vi "Dispense FN - ON - Timer (SubVI).vi"(0 "Settings":T1={"ON Settings"={"Enable Dynamic Setpoint?"=TRUE, "Enable Dynamic Dispense Time?"=TRUE, "Enable Drain Rate Functions"=TRUE, "Dispense Sample Time (s)"=0.1, "Mass Average Samples"=20, "ON Timeout (sec)"=300.0, "1st Setpoint (% of Target)"=90.0, "2nd Setpoint (% of Target)"=95.0, "3rd Setpoint (% of Target)"=100.0, "Measure Dispense Delay (sec)"=10.0, "Minimum Spray Time (s)"=2.0, "Pump Reverse Time (s)"=10.0}, "OFF Settings"={"Drain Sample Time (s)"=0.1, "Drain Rate Ave Size"=100, "Drain Rate Limits (± g/sec)"=100.0, "Level Slope Range (± g/sec)"=0.05, "OFF Timeout (sec)"=300.0, "Near SP Slope Level (± g/sec)"=0.005, "Near Setpoint Threshold (%)"=99.0}, "Overshoot Settings"={"Time Limit (s)"=30.0, "Container MAX (g)"=1500.0, "Max FILL Slope (+/- g/sec)"=100.0, "% Overshot to Enable (>)"=3.0}, "FILL Timeout (s)"=300.0, "Full \nSettle Time (s)"=30.0, "Pre-Hydrate \nSpray Time (s)"=0.0, "Pre-Hydrate \nWait Time (s)"=10.0, "m Value "=1.0, "b Value"=0.0, "Enable Overshoot Adjust?"=FALSE} {"ON Settings"."Pump Reverse Time (s)" min=0.0 max=60.0; "OFF Settings"."Near SP Slope Level (± g/sec)" format="%.3g"; "OFF Settings"."Level Slope Range (± g/sec)" format="%.3g"}, 5 "Reset":bool) -> (14 "Elapsed Time (s)":dbl, 15 "ON Timeout (s)":dbl, 17 "Min Spray Complete?":bool, 18 "Measure Delay Complete?":bool, 19 "Max Spray Complete?":bool)   [LabVIEW 2011]
panel:
  # "ONLY ADJUST\nBOLD VALUES!"
  # "Corrected Mass = SDC Mass * m + b"
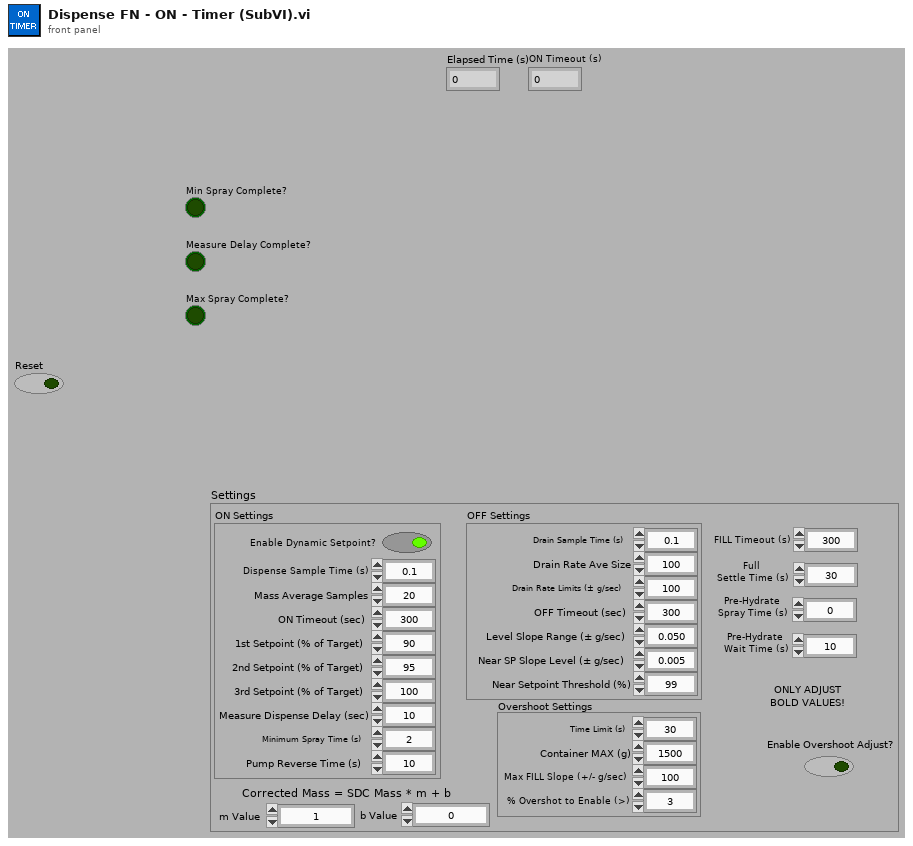
[diagram p1: front panel]
types:
  T1 = cluster{"ON Settings":cluster{"Enable Dynamic Setpoint?":bool, "Enable Dynamic Dispense Time?":bool, "Enable Drain Rate Functions":bool, "Dispense Sample Time (s)":dbl, "Mass Average Samples":i32, "ON Timeout (sec)":dbl, "1st Setpoint (% of Target)":dbl, "2nd Setpoint (% of Target)":dbl, "3rd Setpoint (% of Target)":dbl, "Measure Dispense Delay (sec)":dbl, "Minimum Spray Time (s)":dbl, "Pump Reverse Time (s)":dbl}, "OFF Settings":cluster{"Drain Sample Time (s)":dbl, "Drain Rate Ave Size":i32, "Drain Rate Limits (± g/sec)":dbl, "Level Slope Range (± g/sec)":dbl, "OFF Timeout (sec)":dbl, "Near SP Slope Level (± g/sec)":dbl, "Near Setpoint Threshold (%)":dbl}, "Overshoot Settings":cluster{"Time Limit (s)":dbl, "Container MAX (g)":dbl, "Max FILL Slope (+/- g/sec)":dbl, "% Overshot to Enable (>)":dbl}, "FILL Timeout (s)":dbl, "Full \nSettle Time (s)":dbl, "Pre-Hydrate \nSpray Time (s)":dbl, "Pre-Hydrate \nWait Time (s)":dbl, "m Value ":dbl, "b Value":dbl, "Enable Overshoot Adjust?":bool}
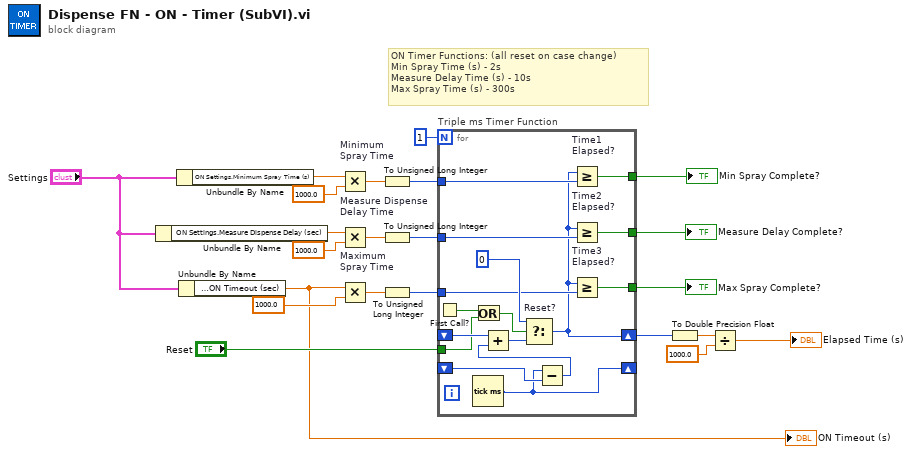
[diagram p0: block diagram]
diagram:
  # "ON Timer Functions: (all reset on case change)\nMin Spray Time (s) - 2s\nMeasure Delay Time (s) - 10s\nMax Spray Time (s) - 300s"
  n1 = Unbundle By Name("Settings") -> ("ON Settings.Measure Dispense Delay (sec)"=w4:dbl)
  n2 = Unbundle By Name("Settings") -> ("ON Settings.Minimum Spray Time (s)"=w3:dbl)
  n3 = Unbundle By Name("Settings") -> ("ON Settings.ON Timeout (sec)"=w5:dbl)
  "ON Timeout (s)" <- w5
  n4 = Multiply "Minimum\nSpray Time"(x=w3, y=1000.0) -> (x*y=w8:dbl)
  n5 = Multiply "Measure Dispense\nDelay Time"(x=w4, y=1000.0) -> (x*y=w13:dbl)
  n6 = Multiply "Maximum\nSpray Time"(x=w5, y=1000.0) -> (x*y=w16:dbl)
  n7 = To Unsigned Long Integer(number=w8) -> (unsigned 32bit integer=w9:u32)
  n8 = To Unsigned Long Integer(number=w13) -> (unsigned 32bit integer=w14:u32)
  n9 = To Unsigned Long Integer(number=w16) -> (unsigned 32bit integer=w17:u32)
  n10 = for "Triple ms Timer Function" {
    N: 1 -> [_]
    shift-right: [w37] -> _
    shift-left: _ -> [w38]
    tunnel: [w36] -> w21
    tunnel: w14 -> [w35]
    shift-right: [w25] -> w19
    shift-left: _ -> [w32]
    tunnel: w9 -> [w31]
    tunnel: [w30] -> w11
    tunnel: w17 -> [w29]
    tunnel: [w28] -> w22
    tunnel: "Reset" -> [w23]
    n11 = First Call?() -> (First Call?: T/F=w24:bool)
    n12 = Tick Count (ms)() -> (millisecond timer value=w37:u32)
    n13 = Or(x=w24, y=w23) -> (x .or. y?=w27:bool)
    n14 = Subtract(x=w37, y=w38) -> (x-y=w26:u32)
    n15 = Add(x=w32, y=w26) -> (x+y=w34:u32)
    n16 = Select "Reset?"(t=u32 0, s=w27, f=w34) -> (s? t:f=w25:u32)
    n17 = Greater Or Equal? "Time1\nElapsed?"(x=w25, y=w31) -> (x >= y?=w30:bool)
    n18 = Greater Or Equal? "Time2\nElapsed?"(x=w25, y=w35) -> (x >= y?=w36:bool)
    n19 = Greater Or Equal? "Time3\nElapsed?"(x=w25, y=w29) -> (x >= y?=w28:bool)
  }
  "Min Spray Complete?" <- w11
  "Measure Delay Complete?" <- w21
  "Max Spray Complete?" <- w22
  n20 = To Double Precision Float(number=w19) -> (double precision float=w18:dbl)
  n21 = Divide(x=w18, y=1000.0) -> (x/y=→"Elapsed Time (s)":dbl)
